vi "OFDM-SIM匹配滤波.vi"(2 "error in (no error)":errorcluster, 3 "input complex waveform":cluster{"t0":dbl, "dt":dbl, "Y":cdb[]}, 4 "?":T1={"过采样因子"=20.0, "脉冲成形参数"={"调制类型"=enum."PSK", "脉冲成形滤波器"=enum."Raised Cosine", "滤波器参数"=0.5, "滤波长度 (码元)"=8.0}, "载波数"=128, "总比特数"=25600, "循环次数"=100, "信噪比门限/dB"=50, "M-QAM (16)"=4} {"脉冲成形参数"."滤波器参数" format="%.2f"}) -> (0 "error out":errorcluster, 1 "output complex waveform":cluster{"t0":dbl, "dt":dbl, "Y":cdb[]})   [LabVIEW 2018]
uses:
  <vilib>/Analysis/2dsp.llb/Decimate (single shot, CDB).vi
  <vilib>/addons/Modulation/Analog/support/mod_Set Error Source.vi
  <vilib>/addons/Modulation/Digital/Support/Common/Validators/mod_Generate Filter Coefficients Validate.vi
  <vilib>/addons/Modulation/Digital/General/subVIs/mod_Generate Filter Coefficients.vi
  <vilib>/addons/Modulation/Digital/General/MT Apply Matched Filter (Generic).vi
  <vilib>/addons/Modulation/Digital/General/MT Align to Ideal Symbols (Generic).vi
  <vilib>/addons/Modulation/niDMT.lvlib
  <vilib>/Analysis/NI_AALPro.lvlib
panel:
  out "大小":i32
  out "alignment offset":dbl
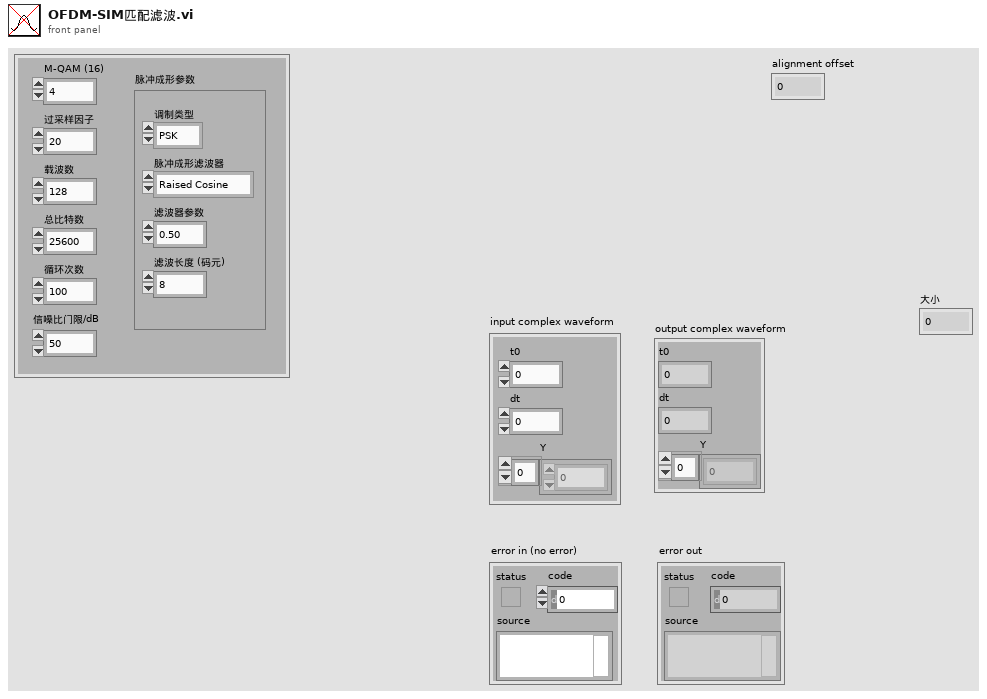
[diagram p1: front panel]
types:
  T1 = cluster{"过采样因子":dbl, "脉冲成形参数":cluster{"调制类型":enum16{"FSK", "PSK", "QAM", "MSK", "PAM", "ASK", "CPM"}, "脉冲成形滤波器":enum16{"none", "Raised Cosine", "Root Raised Cos", "Gaussian"}, "滤波器参数":dbl, "滤波长度 (码元)":dbl}, "载波数":i32, "总比特数":i32, "循环次数":i32, "信噪比门限/dB":i32, "M-QAM (16)":i32}
  T2 = cluster{"调制类型":enum16{"FSK", "PSK", "QAM", "MSK", "PAM", "ASK", "CPM"}, "脉冲成形滤波器":enum16{"none", "Raised Cosine", "Root Raised Cos", "Gaussian"}, "滤波器参数":dbl, "滤波长度 (码元)":dbl}
  T3 = enum16{"FSK", "PSK", "QAM", "MSK", "PAM", "ASK", "CPM"}
  T4 = enum16{"none", "Raised Cosine", "Root Raised Cos", "Gaussian"}
  T5 = typedef "niAMT.lvlib/Complex Data Waveform.ctl" = cluster{"t0":dbl, "dt":dbl, "Y":cdb[]}
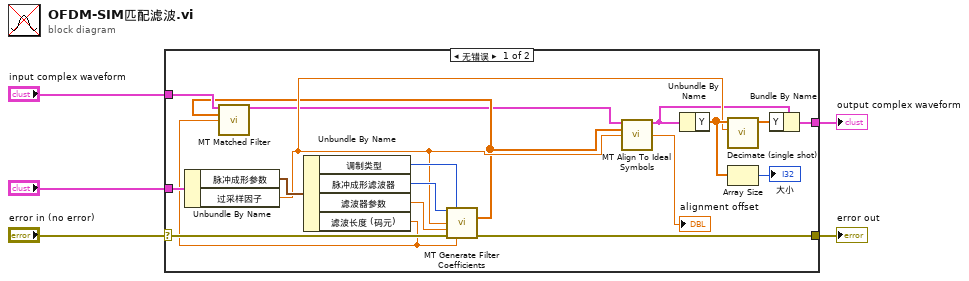
[diagram p0: block diagram]
diagram:
  n1 = case shown="无错误" "error in (no error)" {
    selector: "error in (no error)" -> [w18 w24]
    tunnel: "?" -> [w23 _]
    tunnel: "input complex waveform" -> [w9 _]
    tunnel: [w17 w24] -> w3
    tunnel: [w12 _] -> w2
    frame No Error {
      n2 = Unbundle By Name(w23) -> ("脉冲成形参数"=w22:T2, "过采样因子"=w11:dbl)
      n3 = Unbundle By Name(w22) -> ("调制类型"=w21:T3, "脉冲成形滤波器"=w20:T4, "滤波器参数"=w19:dbl, "滤波长度 (码元)"=w7:dbl)
      n4 = call <vilib>:"MT Generate Filter Coefficients.vi"("pulse shaping filter (none)"=w20, "modulation type"=w21, "matched samples per symbol (16)"=w11, "filter parameter"=w19, "error in (no error)"=w18, "filter length (symbols)"=w7) -> ("matched filter coefficients"=w8:dbl[], "error out"=w17:errorcluster)  [unwired: 7 in, 1 out]
      n5 = call-poly <vilib>:"MT Matched Filter.vi"("input complex waveform"=w9, "matched filter coefficients"=w8, "samples per symbol (16)"=w7) -> ("output complex waveform"=w6:T5)  [unwired: 11 in, 1 out]
      n6 = call-poly <vilib>:"MT Align To Ideal Symbols.vi"("input complex waveform"=w6, "matched filter coefficients"=w8, "samples per symbol (16)"=w11) -> ("output complex waveform"=w10:T5, "waveform alignment offset (samples)"=→"alignment offset":dbl)  [unwired: 10 in, 1 out]
      n7 = Unbundle By Name(w10) -> ("Y"=w14:cdb[])
      n8 = call-poly <vilib>:"Decimate (single shot).vi"("decimating factor"=w11, "X"=w14) -> ("Decimated Array"=w15:cdb[])  [unwired: 8 in, 1 out]
      n9 = Array Size(array=w14) -> (size(s)=→"大小":i32)
      n10 = Bundle By Name(cluster=w10, "Y"=w15) -> (w12:T5)
    }
    frame Error {
    }
  }
  "error out" <- w3
  "output complex waveform" <- w2
